vi "GetSettings.vi"(8 "error in (no error)":errorcluster, 10 "SettingsToRetrieve":variant, 11 "ChromaPowerSupply in":refnum<class "ChromaPowerSupply.lvclass">) -> (0 "error out":errorcluster, 1 "DeviceConfig&Meas":variant, 2 "RetrievedSettings":variant, 3 "ChromaPowerSupply Out":refnum<class "ChromaPowerSupply.lvclass">)   [LabVIEW 2018, in "AcPwrPlugins.lvlib" / "ChromaPowerSupply.lvclass"]
doc: "This VI retrieves the instrument properties."
uses:
  ChromaPowerSupply.lvclass
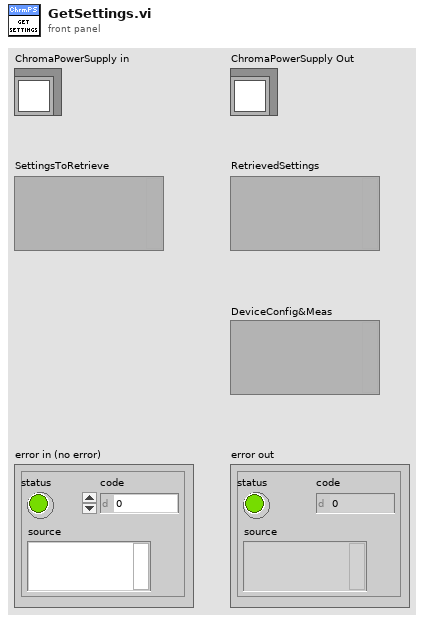
[diagram p1: front panel]
types:
  T1 = typedef "AcPwrPlugins.lvlib/ChromaPowerSupply.lvclass/Measurements.ctl" = cluster{"Handle":string, "Name":string, "Enabled":bool, "Measurement Value":dbl, "btnMeasFetch":bool, "ProtectionStatusString":string, "Measurement Type":enum16{"Voltage (V)", "Current (A)", "Power (W)"}}[]
  T2 = typedef "AcPwrPlugins.lvlib/ChromaPowerSupply.lvclass/Device(s)Settings.ctl" = cluster{"Phases":cluster{"Handle":string, "Instrument Options":string, "id query (T)":bool, "reset device (T)":bool, "Timing":cluster{"TimingOn":enum16{""}, "Hours":u32, "Minutes":u32, "Seconds":dbl, "CutoffVoltage":dbl}, "Connected":bool, "Output Mode":enum16{"Voltage (DC)", "Current (DC)"}, "Voltage":dbl, "Current":dbl, "Voltage Limit":dbl, "Current Limit":dbl}[], "MeasName":string}
  T3 = cluster{"xml string":string, "xml string":string}
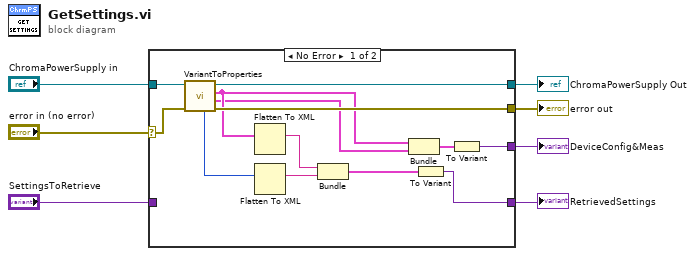
[diagram p0: block diagram]
diagram:
  n1 = case shown="No Error" "error in (no error)" {
    selector: "error in (no error)" -> [w20 w22]
    tunnel: "ChromaPowerSupply in" -> [w19 w23]
    tunnel: [w18 w23] -> w6
    tunnel: [w12 w22] -> w1
    tunnel: "SettingsToRetrieve" -> [_ w21]
    tunnel: [w13 w21] -> w2
    tunnel: [w11 _] -> w5
    frame No Error {
      n2 = call-dynamic "VariantToProperties.vi"("error in (no error)"=w20, "ChromaPowerSupply in"=w19) -> ("error out"=w12:errorcluster, "Measurements"=w9:T1, "Device Settings"=w10:T2, "ChromaPowerSupply out"=w18:refnum<class "ChromaPowerSupply.lvclass">, "Measurement Refresh Time (ms)"=w16:u32)  [unwired: 5 in]
      n3 = Flatten To XML(anything=w10) -> (xml string=w15:string)
      n4 = Flatten To XML(anything=w16) -> (xml string=w14:string)
      n5 = Bundle("xml string"=w15, "xml string"=w14) -> (w17:T3)  [unwired: 1 in]
      n6 = Bundle("Device Settings"=w10, "Measurements"=w9) -> (w8:cluster{"Device Settings":T2, "Measurements":T1})  [unwired: 1 in]
      n7 = To Variant(anything=w17) -> (Variant=w13:variant)
      n8 = To Variant(anything=w8) -> (Variant=w11:variant)
    }
    frame Error {
    }
  }
  "error out" <- w1
  "ChromaPowerSupply Out" <- w6
  "RetrievedSettings" <- w2
  "DeviceConfig&Meas" <- w5
